vi "RetaInimigoBolaUsandoOrientacao.vi"(0 "Y quina":dbl format="%#_13g", 4 "Goal Width":u32, 5 "Field length":u32, 7 "Meio?":bool=TRUE, 8 "Orientação inimigo":dbl format="%#_13g", 10 "Y bola":dbl format="%#_13g", 11 "X bola":dbl format="%#_13g") -> (1 "Orientação goleiro":dbl format="%#_13g", 2 "Y golerio":dbl format="%#_13g", 3 "X goleiro":dbl format="%#_13g")   [LabVIEW 2017]
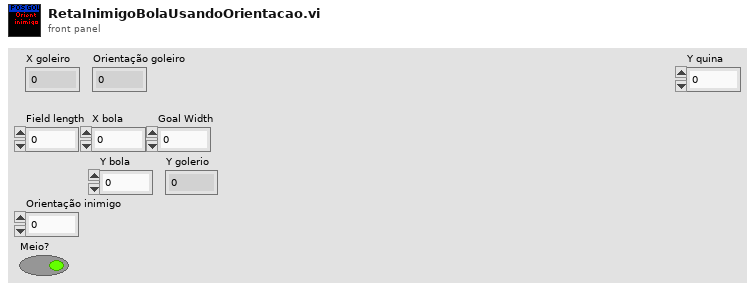
[diagram p1: front panel]
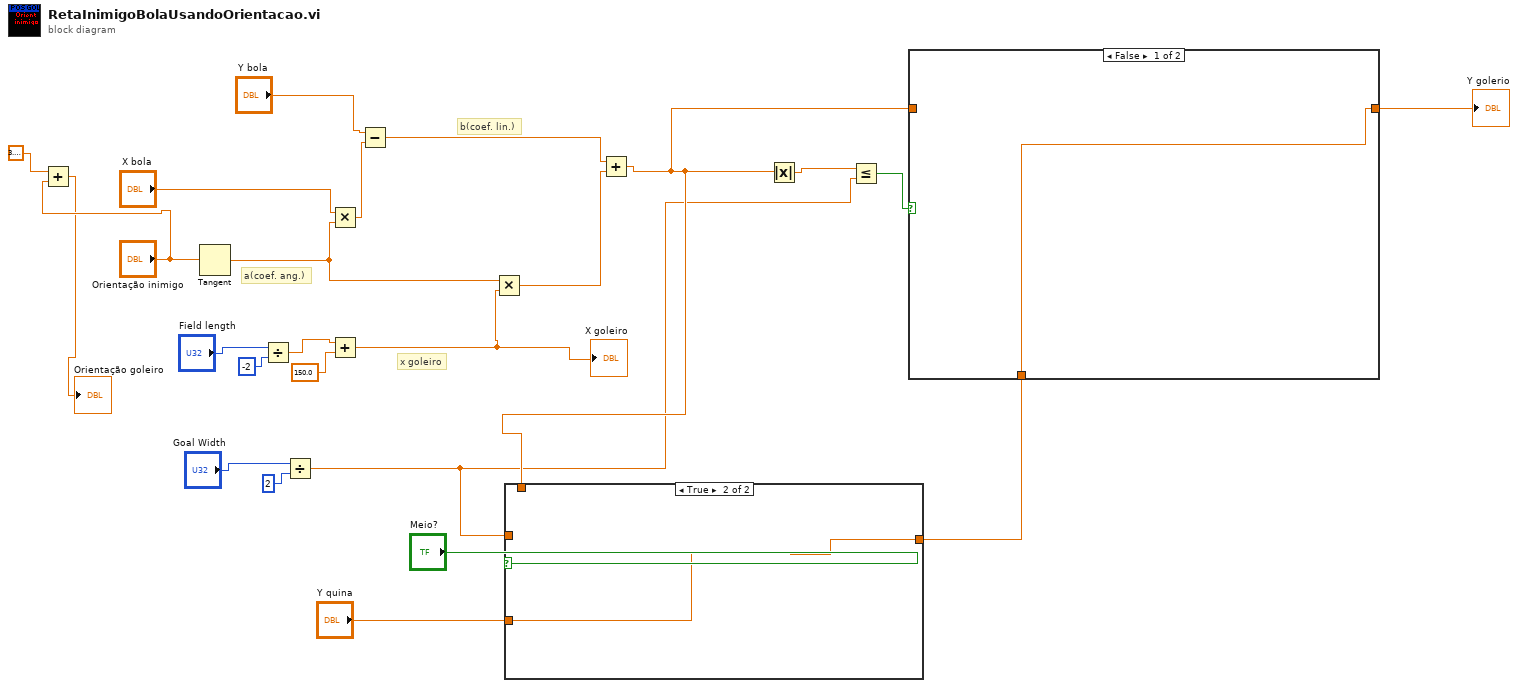
[diagram p0: block diagram]
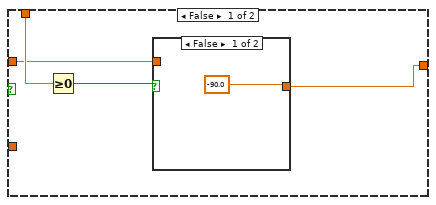
[diagram p2: hidden frame]
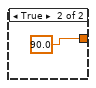
[diagram p3: hidden frame]
diagram:
  # "b(coef. lin.)"
  # "x goleiro"
  # "a(coef. ang.)"
  n1 = Add(x=3.141592653589793, y="Orientação inimigo") -> (x+y=→"Orientação goleiro":dbl)
  n2 = Tangent(1:"Orientação inimigo") -> (0:w17:dbl)
  n3 = Divide(x="Field length", y=-2) -> (x/y=w19:dbl)
  n4 = Divide(x="Goal Width", y=2) -> (x/y=w6:dbl)
  n5 = Multiply(x="X bola", y=w17) -> (x*y=w22:dbl)
  n6 = Add(x=w19, y=150.0 ("x+y")) -> (x+y=w2:dbl)
  "X goleiro" <- w2
  n7 = Subtract(x="Y bola", y=w22) -> (x-y=w16:dbl)
  n8 = Multiply(x=w17, y=w2) -> (x*y=w15:dbl)
  n9 = Add(x=w16, y=w15) -> (x+y=w7:dbl)
  n10 = case shown="True" "Meio?" {
    tunnel: [w25 w31] -> w8
    tunnel: w7 -> [w28 _]
    tunnel: w6 -> [w26 _]
    tunnel: "Y quina" -> [_ w31]
    frame False {
      n11 = Greater Or Equal To 0?(x=w28) -> (x >= 0?=w27:bool)
      n12 = case shown="False" w27 {
        tunnel: w26 -> [_ _]
        tunnel: [-90.0 ("y") 90.0 ("y")] -> w25
        frame False {
        }
        frame True {
        }
      }
    }
    frame True {
    }
  }
  n13 = Absolute Value(x=w7) -> (abs(x)=w12:dbl)
  n14 = Less Or Equal?(x=w12, y=w6) -> (x <= y?=w11:bool)
  n15 = case shown="False" w11 {
    tunnel: [w32 w33] -> w9
    tunnel: w7 -> [_ w33]
    tunnel: w8 -> [w32 _]
    frame False {
    }
    frame True {
    }
  }
  "Y golerio" <- w9
